vi "Database_Init.vi"(2 "error in (no error)":errorcluster, 3 "object in":refnum<class "Database.lvclass">) -> (0 "error out":errorcluster, 1 "object out":refnum<class "Database.lvclass">)   [LabVIEW 2015, in "Database.lvlib" / "Database.lvclass"]
uses:
  Database.lvclass
  Database.lvclass/Database.ctl
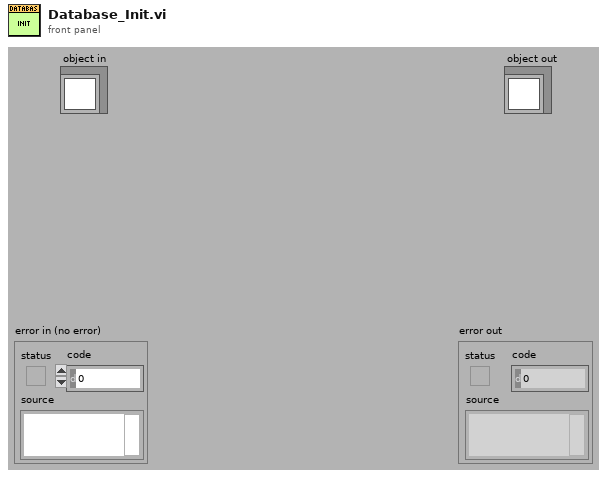
[diagram p1: front panel]
types:
  T1 = enum16{"open", "replace", "create", "open or create", "replace or create", "replace or create with confirmation"}
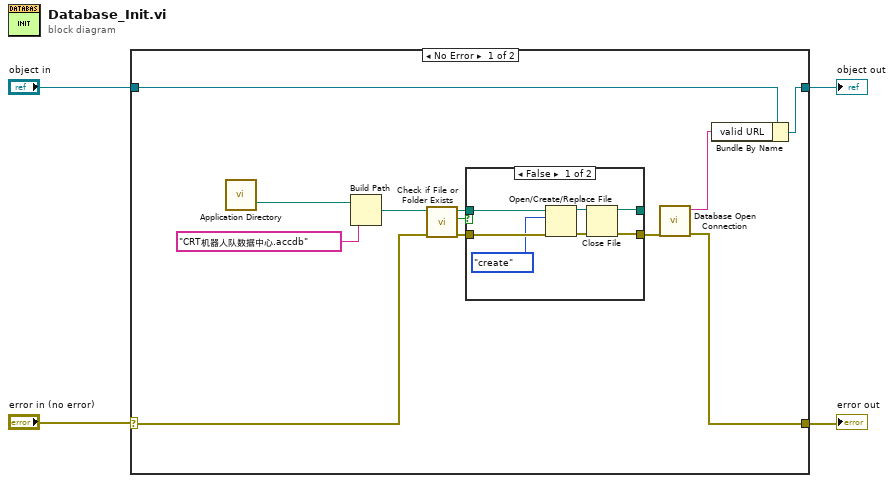
[diagram p0: block diagram]
diagram:
  n1 = case shown="No Error" "error in (no error)" {
    selector: "error in (no error)" -> [w13 w26]
    tunnel: "object in" -> [w7 w27]
    tunnel: [w5 w27] -> w3
    tunnel: [w8 w26] -> w1
    frame No Error {
      n2 = call <vilib>:"Application Directory.vi"() -> ("Application Directory"=w16:path)
      n3 = Build Path(base path=w16, name or relative path="CRT机器人队数据中心.accdb") -> (appended path=w14:path)
      n4 = call <vilib>:"Check if File or Folder Exists.vi"("error in (no error)"=w13, "path"=w14) -> ("error out"=w10:errorcluster, "file or folder exists?"=w12:bool, "dup path"=w11:path)  [unwired: 7 in]
      n5 = case shown="False" w12 {
        tunnel: w11 -> [w23 w25]
        tunnel: w10 -> [w22 w24]
        tunnel: [w18 w25] -> _
        tunnel: [w17 w24] -> w9
        frame False {
          n6 = Open/Create/Replace File(file path (use dialog)=w23, error in=w22, operation (0:open)=T1."create") -> (refnum out=w20:refnum<file>, error out=w19:errorcluster)  [unwired: 3 in, 1 out]
          n7 = Close File(refnum=w20, error in=w19) -> (path=w18:path, error out=w17:errorcluster)
        }
        frame True {
          # "It has exit!"
        }
      }
      n8 = call "Database Open Connection.vi"("error in"=w9) -> ("error out"=w8:errorcluster, "valid URL"=w6:string)  [unwired: 9 in]
      n9 = Bundle By Name(cluster=w7, "valid URL"=w6) -> (w5:refnum<class "Database.lvclass">)
    }
    frame Error {
    }
  }
  "object out" <- w3
  "error out" <- w1
